vi "UDP_Server.vi"() -> ()   [LabVIEW 2020]
panel:
  in  "Puerto de Destino":u16
  in  "stop":bool
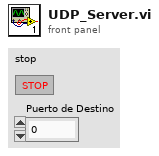
[diagram p1: front panel]
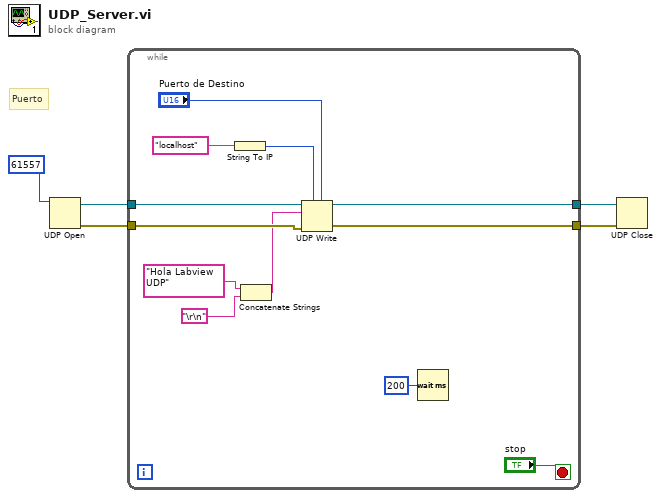
[diagram p0: block diagram]
diagram:
  # "Puerto"
  n1 = UDP Open(11:u16 61557 ("port")) -> (port=w4:refnum<k16>, 0:w3:errorcluster)  [unwired: 4 in, 1 out]
  n2 = while {
    tunnel: w4 -> [w16]
    tunnel: w3 -> [w15]
    tunnel: [w8] -> w2
    tunnel: [w7] -> w1
    stop <- "stop" stop-if-true
    n3 = String To IP(1:"localhost") -> (0:w14:u32)
    n4 = Concatenate Strings("Hola Labview UDP", "\r\n") -> (w10:string)
    n5 = UDP Write(address=w14, port or service name="Puerto de Destino", connection ID=w16, data in=w10, 8:w15) -> (error out=w7:errorcluster, 3:w8:refnum<k16>)  [unwired: 1 in]
    n6 = Wait (ms)(milliseconds to wait=u32 200) -> ()  [unwired: 1 out]
  }
  n7 = UDP Close(connection ID=w2, 8:w1) -> ()  [unwired: 2 out]
